vi "get_device_info.vi"() -> ()   [LabVIEW 2010]
doc: "This VI queries the system information for the device names, product info, and serial number of any National Instruments product installed on your system.\n\nThis VI uses the NI-DAQmx driver software."
uses:
  Program Files/National Instruments/LabVIEW 2010/resource/objmgr/daqmx.rc
panel:
  out "Table":string[][](table)
  # "This VI queries the system information for the device names, product info, and serial \nnumber of any National Instruments product installed on your system.\n\nThis VI uses the NI-DAQmx driver software."
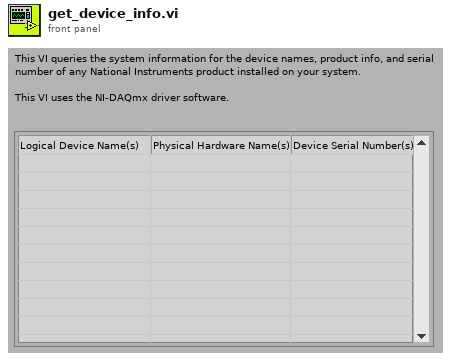
[diagram p1: front panel]
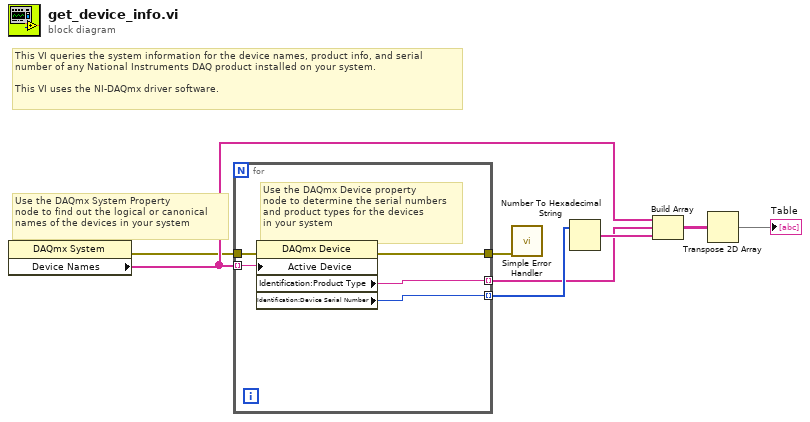
[diagram p0: block diagram]
diagram:
  # "This VI queries the system information for the device names, product info, and serial \nnumber of any National Instruments DAQ product installed on your system.\n\nThis VI uses the NI-DAQmx driver software."
  # "Use the DAQmx System Property\nnode to find out the logical or canonical\nnames of the devices in your system"
  n1 = property class="DAQmx System"() -> (error out=w2:errorcluster, "Device Names"=w3:tag[])  [unwired: 2 in, 1 out]
  n2 = for {
    tunnel: w3 -> [w13] mode=indexing
    tunnel: [w12] -> w6 mode=indexing
    tunnel: [w11] -> w8 mode=indexing
    tunnel: w2 -> [w10]
    tunnel: [w9] -> w1
    # "Use the DAQmx Device property\nnode to determine the serial numbers\nand product types for the devices\nin your system"
    n3 = property class="DAQmx Device"(error in=w10, "Active Device"=w13) -> (error out=w9:errorcluster, "Identification:Product Type"=w12:string, "Identification:Device Serial Number"=w11:u32)  [unwired: 1 in, 1 out]
  }
  n4 = call <vilib>:"Simple Error Handler.vi"("error in (no error)"=w1) -> ()  [unwired: 4 in, 5 out]
  n5 = Number To Hexadecimal String(2:w8) -> (0:w7:string[])  [unwired: 1 in]
  n6 = Build Array(w3, w6, w7) -> (w5:string[][])
  n7 = Transpose 2D Array(2D array=w5) -> (transposed array=→"Table":string[][])
